vi "Tick count to time stamp.vi"(11 "millisecond timer value in":u32 format="%x") -> (2 "current time":timestamp, 3 "time stamp":timestamp)   [LabVIEW 2015]
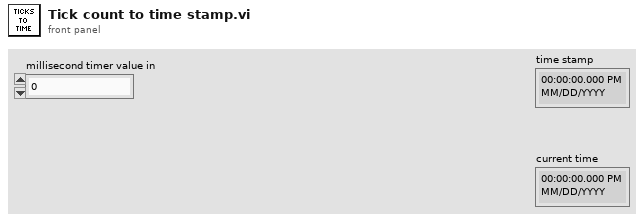
[diagram p1: front panel]
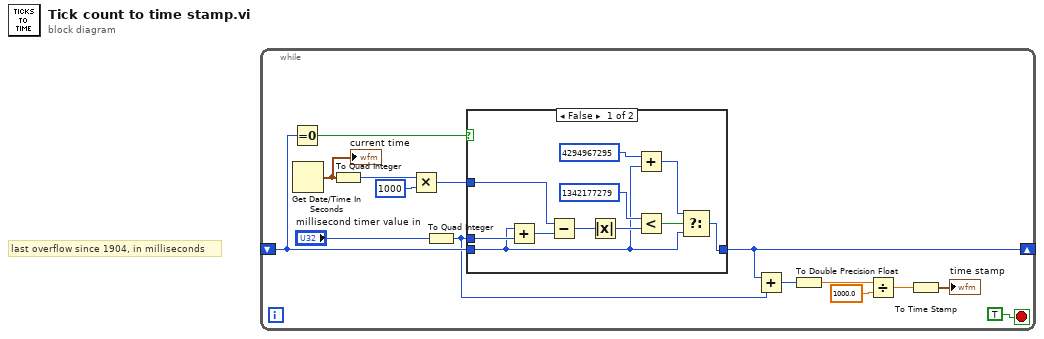
[diagram p0: block diagram]
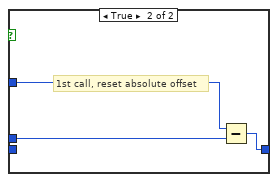
[diagram p2: hidden frame]
diagram:
  # "last overflow since 1904, in milliseconds"
  n1 = while {
    shift-right: [w2] -> _
    shift-left: _ -> [w14]
    stop <- TRUE stop-if-true
    n2 = Equal To 0?(x=w14) -> (x = 0?=w15:bool)
    n3 = Get Date/Time In Seconds() -> (seconds since 1Jan1904=w1:timestamp)
    "current time" <- w1
    n4 = To Quad Integer(1:w1) -> (0:w5:i64)
    n5 = Multiply(x=w5, y=i64 1000) -> (x*y=w4:i64)
    n6 = To Quad Integer(1:"millisecond timer value in") -> (0:w3:i64)
    n7 = case shown="False" w15 {
      tunnel: [w16 w29] -> w2
      tunnel: w14 -> [w18 _]
      tunnel: w3 -> [w22 w28]
      tunnel: w4 -> [w26 w27]
      frame False {
        n8 = Add(x=w18, y=w22) -> (x+y=w21:i64)
        n9 = Subtract(x=w26, y=w21) -> (x-y=w25:i64)
        n10 = Absolute Value(x=w25) -> (abs(x)=w19:i64)
        n11 = Add(x=i64 4294967295 ("millisecond timer value 2"), y=w18) -> (x+y=w23:i64)
        n12 = Less?(x=i64 1342177279 ("millisecond timer value 2"), y=w19) -> (x < y?=w24:bool)
        n13 = Select(t=w23, s=w24, f=w18) -> (s? t:f=w16:i64)
      }
      frame True {
        # "1st call, reset absolute offset"
        n14 = Subtract(x=w27, y=w28) -> (x-y=w29:i64)
      }
    }
    n15 = Add(x=w2, y=w3) -> (x+y=w12:i64)
    n16 = To Double Precision Float(number=w12) -> (double precision float=w11:dbl)
    n17 = Divide(x=w11, y=1000.0) -> (x/y=w9:dbl)
    n18 = To Time Stamp(1:w9) -> (0:→"time stamp":timestamp)
  }
